vi "Autoshifting.vi"(9 "Throttle":dbl, 11 "Manual Low Gear":bool) -> (3 "Low Gear":bool)   [LabVIEW 2013]
uses:
  Robot Global Data.vi
panel:
  out "Down Accel":cluster{dbl, "Numeric":dbl}(graph)
  out "State":enum16{"Low", "High"}(ring)
  out "Throttle Accel":dbl
  out "Speed":dbl
  out "Timer":u32
  out "Up Throttle Accel?":bool
  out "Up Throttle?":bool
  out "Up Accel?":bool
  out "Up Speed?":bool
  out "Up Timer?":bool
  out "Down Timer?":bool
  out "Down Speed?":bool
  out "Down Throttle?":bool
  out "Down Accel?":bool
  out "Accel":dbl
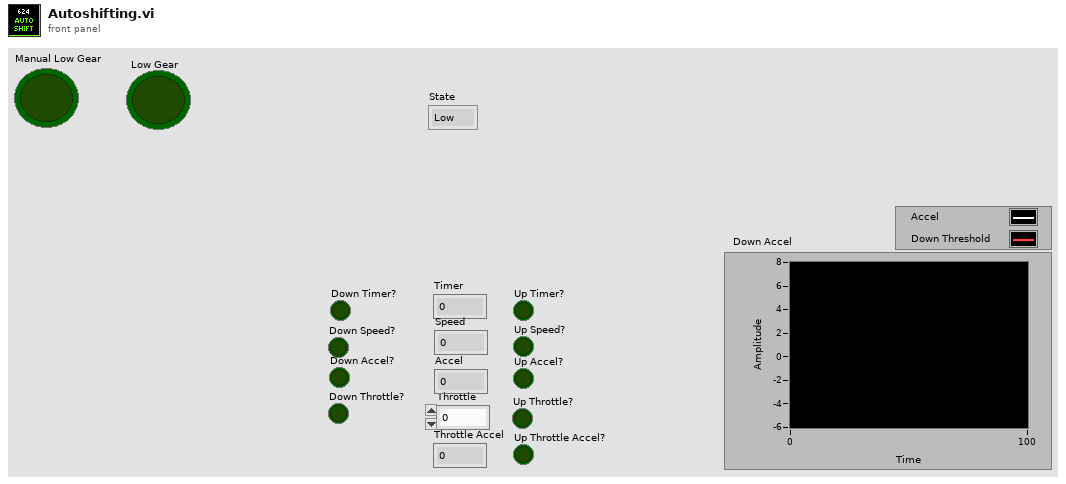
[diagram p1: front panel]
types:
  T1 = typedef "Dashboard UDP Packet.ctl" = cluster{"Camera":T2, "Gyro":T3, "Encoder":T4, "Auto Shift":T5, "Auton":T6, "Drive/Ramp X":dbl, "Drive/Ramp Y":dbl, "Drive/Battery Cutoff":dbl, "Pressure/Compressor Min Voltage":dbl, "Pressure/Compressor Delay":dbl, "Controller/Strafe Correction":bool, "Shooter":T7, "Rollers":T8, "Abort":bool, "Finish":bool}
  T2 = typedef "Camera Controls.ctl" = cluster{"Camera/View Angle X":dbl, "Camera/Goal Track Timeout":dbl, "Camera/View Angle Y":dbl, "Camera/Goal Exposure":dbl, "Camera/Vision Receive Timeout":dbl, "Camera/Offset 1":dbl, "Camera/Offset 2":dbl}
  T3 = typedef "Gyro Controls.ctl" = cluster{"Gyro/Steer Close PID P":dbl, "Gyro/Steer Close PID I":dbl, "Gyro/Steer Close PID D":dbl, "Gyro/Steer Close PID min":dbl, "Gyro/Steer Close PID max":dbl, "Gyro/Steer PID P":dbl, "Gyro/Steer PID I":dbl, "Gyro/Steer PID D":dbl, "Gyro/Steer PID min":dbl, "Gyro/Angle Tolerance":dbl, "Gyro/Steer PID max":dbl, "Gyro/Steer Closeness Threshold":dbl}
  T4 = typedef "Encoder Controls.ctl" = cluster{"Encoders/Reset":bool, "Encoders/Omni Constant":dbl, "Encoders/Omni Tick Constant":dbl, "Encoders/Left Constant":dbl, "Encoders/Right Constant":dbl, "Encoders/Right Tick Constant":dbl}
  T5 = typedef "Auto Shift Controls.ctl" = cluster{"AutoShift/Upshift Throttle Accel":dbl, "AutoShift/Speed Threshold":dbl, "AutoShift/Upshift Throttle":dbl, "AutoShift/Upshift Accel":dbl, "AutoShift/Downshift Accel":dbl, "AutoShift/Downshift Throttle":dbl, "AutoShift/Delay":dbl, "AutoShift/Enabled":bool}
  T6 = typedef "Auton Controls.ctl" = cluster{"Auton/Left Shoot X-Coord":dbl, "Auton/Right Shoot X-Coord":dbl, "DistDrive/Distance Stop Threshold":dbl, "DistDrive/Max Stop Speed":dbl, "Auton/Back Piston Time":dbl, "Auton/Manual Hot":bool, "Auton/Manual Hot Right":bool, "Auton/X Distance PID max":dbl, "Auton/X Distance PID min":dbl, "Auton/X Distance PID P":dbl, "Auton/X Distance PID I":dbl, "Auton/X Distance PID D":dbl, "Auton/Y Distance PID max":dbl, "Auton/Y Distance PID min":dbl, "Auton/Y Distance PID P":dbl, "Auton/Y Distance PID I":dbl, "Auton/Y Distance PID D":dbl}
  T7 = typedef "Shooter Controls.ctl" = cluster{"Shooter/Reset Time":dbl, "Shooter/Release Delay":dbl, "Shooter/Pressure Steady Time":dbl, "Shooter/Misfire Delay":dbl, "Shooter/Ball Settle Time":dbl, "Shooter/Line IR Delay":dbl, "Pressure/Upper PSI Time":dbl, "Pressure/Lower PSI Time":dbl, "Shooter/Punch Delay":dbl, "Shooter/Target Pressure":dbl, "Pressure/Line B":dbl, "Pressure/Line M":dbl, "Pressure/Shooter M":dbl, "Pressure/Shooter B":dbl}
  T8 = typedef "Roller Controls.ctl" = cluster{"Roller/Load IRs Verify Time":dbl, "Roller/Center IR Latch Time":dbl, "Roller/Speed Front":dbl, "Roller/Speed Back":dbl, "Roller/Entry Timeout":dbl, "Roller/To Center Timeout":dbl, "Roller/Sustain Time":dbl, "Roller/Verify Center Time":dbl}
  T9 = typedef "Encoder Data.ctl" = cluster{"Avg Distance L/R":dbl, "Avg Speed L/R":dbl, "Left":T10, "Right":T10, "Omni":T10}
  T10 = typedef "Single Encoder Data.ctl" = cluster{"Distance":dbl, "Speed":dbl, "Ticks":dbl}
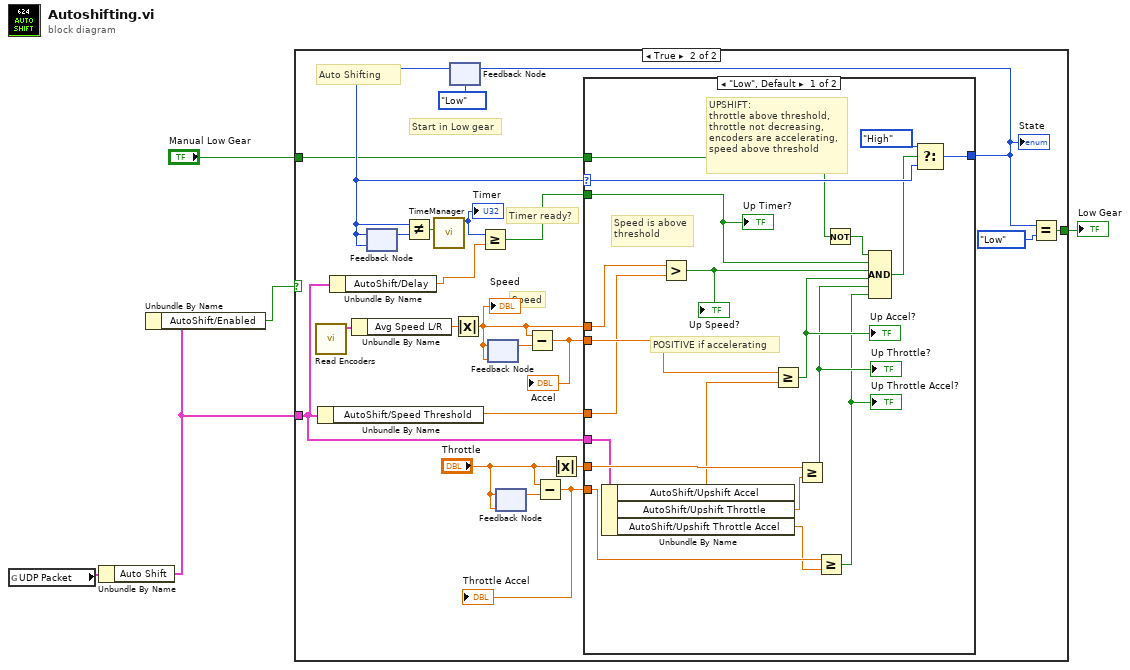
[diagram p0: block diagram]
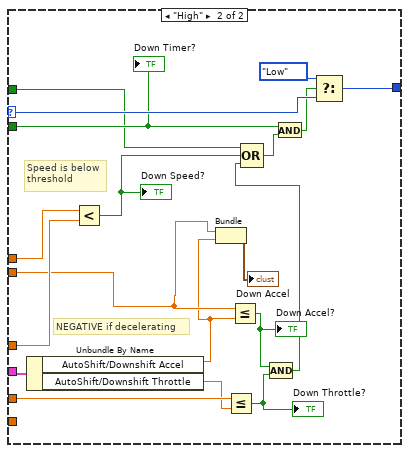
[diagram p3: hidden frame]
diagram:
  n1 = global read "Robot Global Data.vi" "UDP Packet"() -> (w3:T1)
  n2 = Unbundle By Name(w3) -> ("Auto Shift"=w1:T5)
  n3 = Unbundle By Name(w1) -> ("AutoShift/Enabled"=w2:bool)
  n4 = case shown="True" w2 {
    tunnel: [w6 w18] -> w5
    tunnel: "Manual Low Gear" -> [w6 w13]
    tunnel: w1 -> [_ w7]
    frame False {
      # "Manual Shifting"
    }
    frame True {
      # "Auto Shifting"
      # "Timer ready?"
      # "Speed"
      # "Start in Low gear"
      n5 = call "Read Encoders.vi"() -> ("Encoder Data"=w21:T9)  [unwired: 11 in]
      n6 = Unbundle By Name(w7) -> ("AutoShift/Speed Threshold"=w9:dbl)
      n7 = Unbundle By Name(w7) -> ("AutoShift/Delay"=w8:dbl)
      n8 = Unbundle By Name(w21) -> ("Avg Speed L/R"=w22:dbl)
      n9 = feedback #1(enum16{"Low", "High"}."Low") -> (w24:enum16{"Low", "High"})
      n10 = feedback #2(w24) -> (w27:enum16{"Low", "High"})
      n11 = feedback-in #2(w24) -> ()
      n12 = Not Equal?(x=w24, y=w27) -> (x != y?=w28:bool)
      n13 = call "TimeManager.vi"("Reset?"=w28) -> ("Time Since Reset"=w26:u32)  [unwired: 9 in, 1 out]
      "Timer" <- w26
      n14 = Absolute Value(x=w22) -> (abs(x)=w16:dbl)
      "Speed" <- w16
      n15 = Greater Or Equal?(x=w26, y=w8) -> (x >= y?=w25:bool)
      n16 = feedback-in #3(w16) -> ()
      n17 = feedback #3(w16) -> (w17:dbl)
      n18 = feedback #4("Throttle") -> (w15:dbl)
      n19 = feedback-in #4("Throttle") -> ()
      n20 = Subtract(x=w16, y=w17) -> (x-y=w12:dbl)
      "Accel" <- w12
      n21 = Subtract(x="Throttle", y=w15) -> (x-y=w14:dbl)
      "Throttle Accel" <- w14
      n22 = Absolute Value(x="Throttle") -> (abs(x)=w10:dbl)
      n23 = case shown="\"Low\", Default" w24 {
        selector: w24 -> [w46 w65]
        tunnel: w25 -> [w44 w55]
        tunnel: [w47 w66] -> w20
        tunnel: w16 -> [w42 w64]
        tunnel: w9 -> [w41 w62]
        tunnel: w12 -> [w43 w52]
        tunnel: w10 -> [w35 w61]
        tunnel: w14 -> [w39 _]
        tunnel: w13 -> [w33 w54]
        tunnel: w7 -> [w29 w49]
        frame "Low", Default {
          # "UPSHIFT:\nthrottle above threshold,\nthrottle not decreasing,\nencoders are accelerating,\nspeed above threshold"
          # "Speed is above\nthreshold"
          # "POSITIVE if accelerating"
          n24 = Unbundle By Name(w29) -> ("AutoShift/Upshift Accel"=w30:dbl, "AutoShift/Upshift Throttle"=w31:dbl, "AutoShift/Upshift Throttle Accel"=w32:dbl)
          n25 = Greater?(x=w42, y=w41) -> (0:w40:bool)
          "Up Speed?" <- w40
          n26 = Greater Or Equal?(x=w43, y=w30) -> (x >= y?=w38:bool)
          "Up Accel?" <- w38
          n27 = Greater Or Equal?(x=w35, y=w31) -> (x >= y?=w37:bool)
          "Up Throttle?" <- w37
          n28 = Greater Or Equal?(x=w39, y=w32) -> (x >= y?=w36:bool)
          "Up Throttle Accel?" <- w36
          n29 = Not(x=w33) -> (.not. x?=w34:bool)
          n30 = Compound Arithmetic op=AND(w34, w44, w40, w38, w37, w36) -> (w45:bool)
          n31 = Select(t=enum16{"Low", "High"}."High", s=w45, f=w46) -> (s? t:f=w47:enum16{"Low", "High"})
          "Up Timer?" <- w44
        }
        frame "High" {
          # "NEGATIVE if decelerating"
          # "Speed is below\nthreshold"
          n32 = Unbundle By Name(w49) -> ("AutoShift/Downshift Accel"=w51:dbl, "AutoShift/Downshift Throttle"=w50:dbl)
          n33 = Less?(x=w64, y=w62) -> (x < y?=w63:bool)
          "Down Speed?" <- w63
          n34 = Bundle(w52, "AutoShift/Downshift Accel"=w51) -> (→"Down Accel":cluster{dbl, "AutoShift/Downshift Accel":dbl})  [unwired: 1 in]
          n35 = Less Or Equal?(x=w61, y=w50) -> (x <= y?=w59:bool)
          "Down Throttle?" <- w59
          n36 = Less Or Equal?(x=w52, y=w51) -> (x <= y?=w60:bool)
          "Down Accel?" <- w60
          n37 = Compound Arithmetic op=AND(w60, w59) -> (w58:bool)
          n38 = Compound Arithmetic op=OR(w54, w63, w58) -> (w57:bool)
          n39 = And(x=w55, y=w57) -> (x .and. y?=w56:bool)
          n40 = Select(t=enum16{"Low", "High"}."Low", s=w56, f=w65) -> (s? t:f=w66:enum16{"Low", "High"})
          "Down Timer?" <- w55
        }
      }
      "State" <- w20
      n41 = feedback-in #1(w20) -> ()
      n42 = Equal?(x=w20, y=enum16{"Low", "High"}."Low") -> (x = y?=w18:bool)
    }
  }
  "Low Gear" <- w5
